vi "TDMScompress.vi"() -> ()   [LabVIEW 2012]
panel:
  out "Error Array":errorcluster[](array[cluster])
  out "num chans":i32
  out "Num Errors":i32
  out "Compressing":bool
  out "Current File":string
  out "File Index":i32
  out "Size":i32
  out "Filenames":string[](array[string])
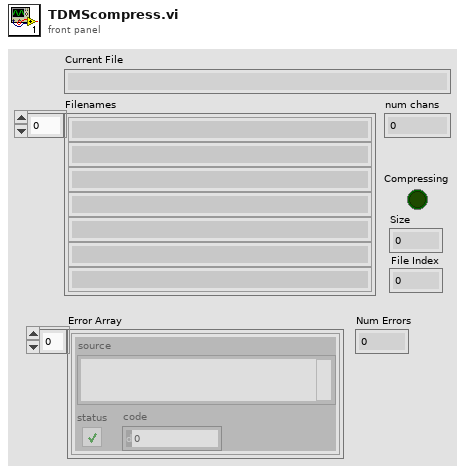
[diagram p1: front panel]
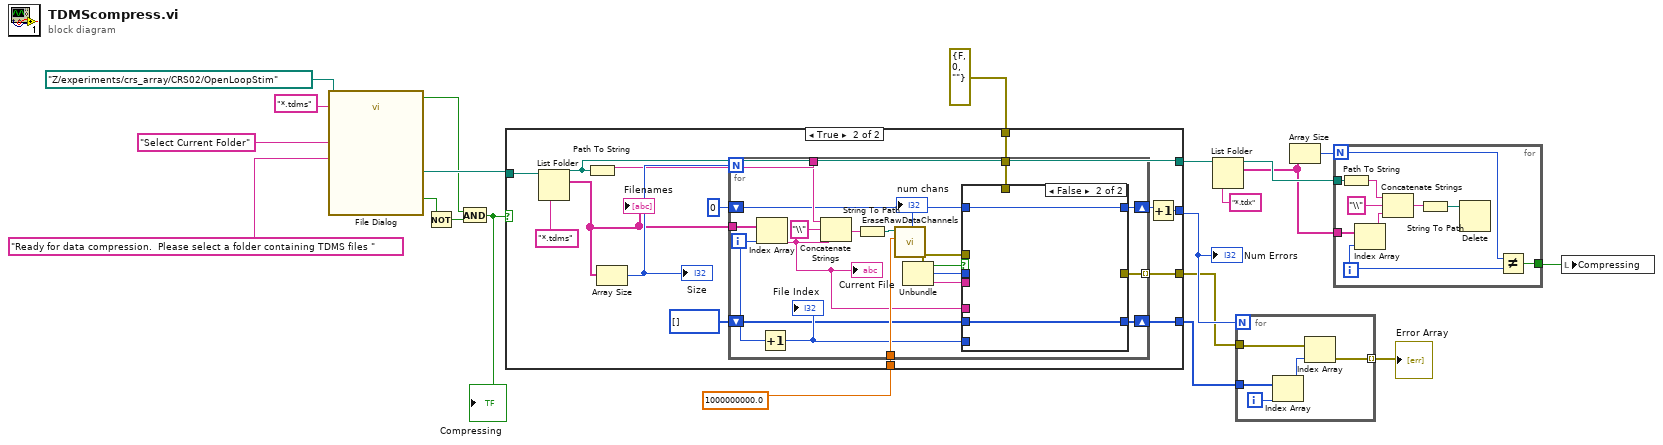
[diagram p0: block diagram]
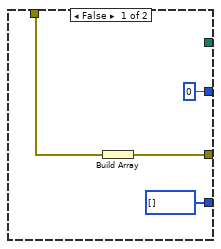
[diagram p2: hidden frame]
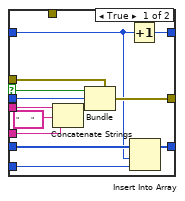
[diagram p3: hidden frame]
diagram:
  n1 = call "File Dialog"("start path"=path "Z:/experiments/crs_array/CRS02/OpenLoopStim", "prompt"="Ready for data compression.  Please select a folder containing TDMS files ", "button label"="Select Current Folder", "pattern (all files)"="*.tdms" ("pattern label")) -> ("selected path"=w21:path, "exists"=w14:bool, "cancelled"=w18:bool)  [unwired: 8 in, 1 out]
  n2 = Not(x=w18) -> (.not. x?=w15:bool)
  n3 = And(x=w14, y=w15) -> (x .and. y?=w16:bool)
  "Compressing" <- w16
  n4 = case shown="True" w16 {
    tunnel: w21 -> [_ w35]
    tunnel: [_ w34] -> w13
    tunnel: 1000000000.0 ("File Limit Size") -> [_ w33]
    tunnel: [0 w30] -> w4
    tunnel: [w23 w29] -> w3
    tunnel: errorcluster {"status"=FALSE, "code"=0, "source"=""} ("output cluster") -> [w24 w28]
    tunnel: [i32[] [] w26] -> w2
    frame False {
      n5 = Build Array(w24) -> (w23:errorcluster[])
    }
    frame True {
      n6 = List Folder(path=w35, pattern="*.tdms") -> (path out=w34:path, filenames=w37:string[])  [unwired: 2 in, 2 out]
      "Filenames" <- w37
      n7 = Path To String(path=w34) -> (string=w36:string)
      n8 = Array Size(array=w37) -> (size(s)=w38:i32)
      "Size" <- w38
      n9 = for {
        N: w38 -> [_]
        tunnel: w37 -> [w59]
        tunnel: w36 -> [w56]
        tunnel: w33 -> [w53]
        shift-right: [w45] -> w31
        shift-left: 0 ("size(s)") -> [w46]
        tunnel: [w44] -> w29 mode=indexing
        tunnel: w28 -> [w43]
        shift-right: [w41] -> w26
        shift-left: i32[] [] -> [w40]
        i -> [w58]
        n10 = Index Array(array=w59, index=w58) -> (element=w48:string)
        "Current File" <- w48
        n11 = Increment(x=w58) -> (x+1=w42:i32)
        "File Index" <- w42
        n12 = Concatenate Strings(w56, "\\" ("string"), w48) -> (w57:string)
        n13 = String To Path(string=w57) -> (path=w54:path)
        n14 = call "EraseRawDataChannels.vi"("File Limit Size"=w53, "TDMS file path in"=w54) -> ("error out"=w47:errorcluster, "num chans"=→"num chans":i32)  [unwired: 6 in, 1 out]
        n15 = Unbundle(w47) -> ("status"=w51:bool, "code"=w50:i32, "source"=w49:string)
        n16 = case shown="False" w51 {
          selector: w51 -> [w72 _]
          tunnel: w50 -> [w66 _]
          tunnel: w49 -> [w71 _]
          tunnel: w48 -> [w61 _]
          tunnel: w47 -> [w69 _]
          tunnel: w46 -> [w64 w74]
          tunnel: [w68 w74] -> w45
          tunnel: [w67 _] -> w44
          tunnel: w43 -> [_ _]
          tunnel: w42 -> [w63 _]
          tunnel: [w62 w73] -> w41
          tunnel: w40 -> [w65 w73]
          frame True {
            n17 = Concatenate Strings(w71, "      " ("string"), w61) -> (w70:string)
            n18 = Bundle(cluster=w69, "status"=w72, "code"=w66, "source"=w70) -> (w67:errorcluster)
            n19 = Increment(x=w64) -> (x+1=w68:i32)
            n20 = Insert Into Array(array=w65, index=w64, new element=w63) -> (w62:i32[])
          }
          frame False {
          }
        }
      }
      n21 = Increment(x=w31) -> (x+1=w30:i32)
    }
  }
  "Num Errors" <- w4
  n22 = List Folder(path=w13, pattern="*.tdx") -> (path out=w11:path, filenames=w9:string[])  [unwired: 2 in, 2 out]
  n23 = for {
    N: w4 -> [_]
    tunnel: w3 -> [w76]
    tunnel: w2 -> [w79]
    tunnel: [w75] -> w1 mode=indexing
    i -> [w78]
    n24 = Index Array(array=w79, index=w78) -> (element=w77:i32)
    n25 = Index Array(array=w76, index=w77) -> (element=w75:errorcluster)
  }
  "Error Array" <- w1
  n26 = Array Size(array=w9) -> (size(s)=w10:i32)
  n27 = for {
    N: w10 -> [w82]
    tunnel: w11 -> [w89]
    tunnel: w9 -> [w86]
    tunnel: [w80] -> w6
    i -> [w81]
    n28 = Path To String(path=w89) -> (string=w87:string)
    n29 = Index Array(array=w86, index=w81) -> (element=w85:string)
    n30 = Concatenate Strings(w87, "\\" ("string"), w85) -> (w84:string)
    n31 = String To Path(string=w84) -> (path=w83:path)
    n32 = Delete(path (use dialog)=w83) -> ()  [unwired: 4 in, 3 out]
    n33 = Not Equal?(x=w82, y=w81) -> (x != y?=w80:bool)
  }
  n34 = local write "Compressing"(w6) -> ()
